vi "GL_MHeaterInput.vi"() -> ()   [LabVIEW 2019]
panel:
  in  "MANUAL HEATER":dbl(slide) caption="AMP" min=0.0 max=5.0 scale=0.0..5.0
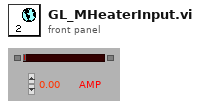
[diagram p1: front panel]
diagram:
